vi "raptor_get_en_face.vi"(8 "error in (no error)":errorcluster, 11 "Image Src":T1) -> (0 "error out":errorcluster, 3 "Image Dst Out":T1)   [LabVIEW 2016]
doc: "Raptor: Returns the current en face image being assembled."
uses:
  <vilib>/vision/Image Controls.llb/IMAQ Image.ctl
  globals/Channel 1 Image Ring.vi
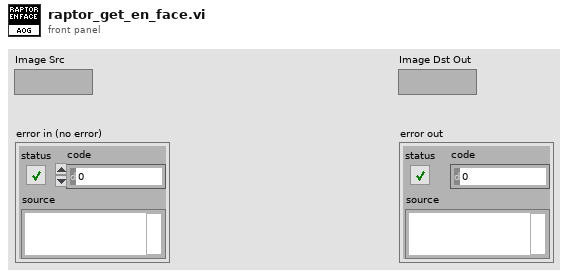
[diagram p1: front panel]
types:
  T1 = typedef "IMAQ Image.ctl" = refnum<image>
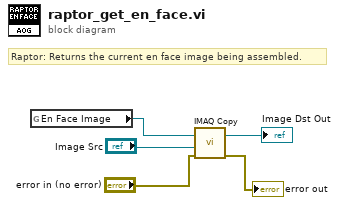
[diagram p0: block diagram]
diagram:
  # "Raptor: Returns the current en face image being assembled."
  n1 = global read "Channel 1 Image Ring.vi" "En Face Image"() -> (w2:T1)
  n2 = call "IMAQ Copy"("error in (no error)"="error in (no error)", "Image Dst"="Image Src", "Image Src"=w2) -> ("error out"=→"error out":errorcluster, "Image Dst Out"=→"Image Dst Out":T1)  [unwired: 3 in]
